vi "SUB_COM1_WR_FindString.vi"(3 "Find this String":string, 4 "write buffer":string, 5 "number of char to read":i32, 6 "VISA resource name":refnum<visa-resource-name>) -> (0 "duplicate VISA resource name":refnum<visa-resource-name>, 1 "Found":bool, 2 "Output String":string)   [LabVIEW 2011]
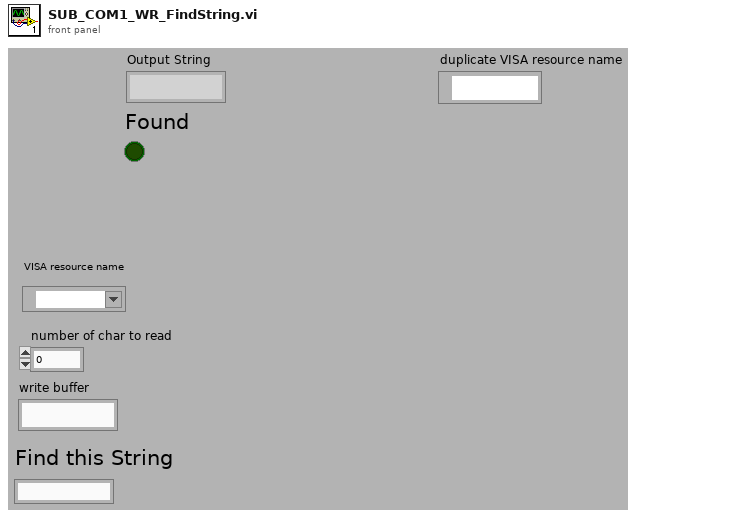
[diagram p1: front panel]
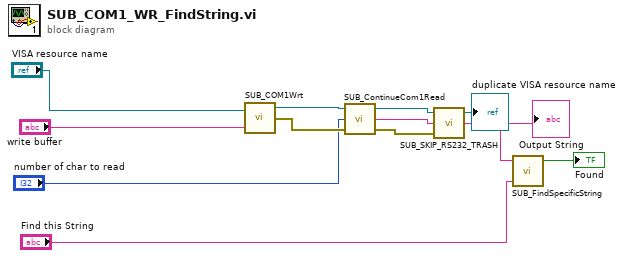
[diagram p0: block diagram]
diagram:
  n1 = call "SUB_COM1Wrt.vi"("VISA resource name"="VISA resource name", "write buffer"="write buffer") -> ("duplicate VISA resource name"=w12:refnum<visa-resource-name>, "error out"=w10:errorcluster)  [unwired: 1 out]
  n2 = call "SUB_ContinueCom1Read.vi"("error out 2"=w10, "Numeric"="number of char to read", "duplicate VISA resource name 2"=w12) -> ("error out"=w9:errorcluster, "String"=w8:string, "duplicate VISA resource name"=w11:refnum<visa-resource-name>)
  n3 = call "SUB_SKIP_RS232_TRASH.vi"("error out 2"=w9, "read buffer"=w8, "duplicate VISA resource name 2"=w11) -> ("String"=w7:string, "duplicate VISA resource name"=→"duplicate VISA resource name":refnum<visa-resource-name>)  [unwired: 1 out]
  "Output String" <- w7
  n4 = call "SUB_FindSpecificString.vi"("Find this String"="Find this String", "String data"=w7) -> ("Found"=→"Found":bool)  [unwired: 2 in, 1 out]
